vi "testing.vi"() -> ()   [LabVIEW 2013]
panel:
  out "Numeric 2":dbl
  in  "Numeric":dbl
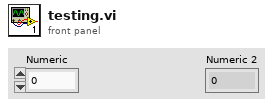
[diagram p1: front panel]
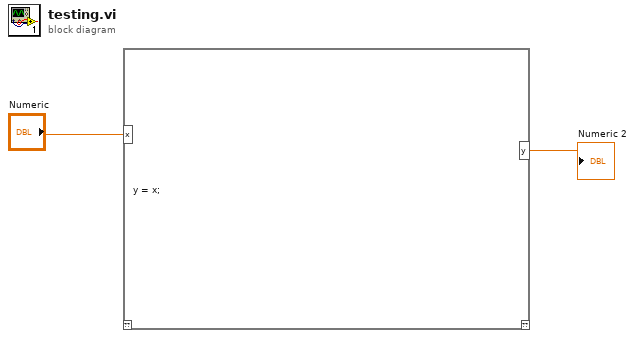
[diagram p0: block diagram]
diagram:
  n1 = script code="y = x;"("x"="Numeric") -> ("y"=→"Numeric 2":dbl)  [unwired: 1 in, 1 out]
